vi "GripperPosition.vi"   [LabVIEW 2016]
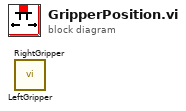
[diagram p0: block diagram]
diagram:
  n1 = call "LeftGripper.vi"() -> ()  [unwired: 4 in, 1 out]
  n2 = call "RightGripper.vi"() -> ()  [unwired: 4 in, 1 out]
